vi "BaudDetect-GetDetectArray.vi"(8 "SAM":u8(ring) caption="采样点:" items=["采样一次", "采样三次"], 9 "SJW":u8(ring)=1 caption="同步跳转宽度:" items=["1TQ"=1, "2TQ"=2, "3TQ"=3, "4TQ"=4], 10 "g_data":T2={"b"=-1.0, "e"=-1.0}, 11 "DetectArray in":cluster{"T0":u8, "T1":u8, "br_selfdef":T1}[](array[cluster]) {"br_selfdef"."PHSEG2" items=["CAN_BIT_1TQ"=1, "CAN_BIT_2TQ"=2, "CAN_BIT_3TQ"=3, "CAN_BIT_4TQ"=4, "CAN_BIT_5TQ"=5, "CAN_BIT_6TQ"=6, "CAN_BIT_7TQ"=7, "CAN_BIT_8TQ"=8]; "br_selfdef"."PHSEG1" items=["CAN_BIT_1TQ"=1, "CAN_BIT_2TQ"=2, "CAN_BIT_3TQ"=3, "CAN_BIT_4TQ"=4, "CAN_BIT_5TQ"=5, "CAN_BIT_6TQ"=6, "CAN_BIT_7TQ"=7, "CAN_BIT_8TQ"=8]; "br_selfdef"."PRSEG" items=["CAN_BIT_1TQ"=1, "CAN_BIT_2TQ"=2, "CAN_BIT_3TQ"=3, "CAN_BIT_4TQ"=4, "CAN_BIT_5TQ"=5, "CAN_BIT_6TQ"=6, "CAN_BIT_7TQ"=7, "CAN_BIT_8TQ"=8]; "br_selfdef"."PHS2_SEL" items=["由相位缓冲段1时间指定", "可编程"]; "br_selfdef"."SAM" items=["采样一次", "采样三次"]; "br_selfdef"."BRP" items=["1"=1, "2"=2, "3"=3, "4"=4, "5"=5, "6"=6, "7"=7, "8"=8, "9"=9, "10"=10, "11"=11, "12"=12, "13"=13, "14"=14, "15"=15, "16"=16, "17"=17, "18"=18, "19"=19, "20"=20, "21"=21, "22"=22, "23"=23, "24"=24, "25"=25, "26"=26, "27"=27, "28"=28, "29"=29, "30"=30, "31"=31, "32"=32, "33"=33, "34"=34, "35"=35, "36"=36, "37"=37, "38"=38, "39"=39, "40"=40, "41"=41, "42"=42, "43"=43, "44"=44, "45"=45, "46"=46, "47"=47, "48"=48, "49"=49, "50"=50, "51"=51, "52"=52, "53"=53, "54"=54, "55"=55, "56"=56, "57"=57, "58"=58, "59"=59, "60"=60, "61"=61, "62"=62, "63"=63, "64"=64]; "br_selfdef"."SJW" items=["1TQ"=1, "2TQ"=2, "3TQ"=3, "4TQ"=4]; "br_selfdef"."SYN(nouse)" items=["CAN_BIT_1TQ"=1]}) -> (3 "DetectArray out":cluster{"T0":u8, "T1":u8, "br_selfdef":T1}[](array[cluster]) {"br_selfdef"."PHSEG2" items=["CAN_BIT_1TQ"=1, "CAN_BIT_2TQ"=2, "CAN_BIT_3TQ"=3, "CAN_BIT_4TQ"=4, "CAN_BIT_5TQ"=5, "CAN_BIT_6TQ"=6, "CAN_BIT_7TQ"=7, "CAN_BIT_8TQ"=8]; "br_selfdef"."PHSEG1" items=["CAN_BIT_1TQ"=1, "CAN_BIT_2TQ"=2, "CAN_BIT_3TQ"=3, "CAN_BIT_4TQ"=4, "CAN_BIT_5TQ"=5, "CAN_BIT_6TQ"=6, "CAN_BIT_7TQ"=7, "CAN_BIT_8TQ"=8]; "br_selfdef"."PRSEG" items=["CAN_BIT_1TQ"=1, "CAN_BIT_2TQ"=2, "CAN_BIT_3TQ"=3, "CAN_BIT_4TQ"=4, "CAN_BIT_5TQ"=5, "CAN_BIT_6TQ"=6, "CAN_BIT_7TQ"=7, "CAN_BIT_8TQ"=8]; "br_selfdef"."PHS2_SEL" items=["由相位缓冲段1时间指定", "可编程"]; "br_selfdef"."SAM" items=["采样一次", "采样三次"]; "br_selfdef"."BRP" items=["1"=1, "2"=2, "3"=3, "4"=4, "5"=5, "6"=6, "7"=7, "8"=8, "9"=9, "10"=10, "11"=11, "12"=12, "13"=13, "14"=14, "15"=15, "16"=16, "17"=17, "18"=18, "19"=19, "20"=20, "21"=21, "22"=22, "23"=23, "24"=24, "25"=25, "26"=26, "27"=27, "28"=28, "29"=29, "30"=30, "31"=31, "32"=32, "33"=33, "34"=34, "35"=35, "36"=36, "37"=37, "38"=38, "39"=39, "40"=40, "41"=41, "42"=42, "43"=43, "44"=44, "45"=45, "46"=46, "47"=47, "48"=48, "49"=49, "50"=50, "51"=51, "52"=52, "53"=53, "54"=54, "55"=55, "56"=56, "57"=57, "58"=58, "59"=59, "60"=60, "61"=61, "62"=62, "63"=63, "64"=64]; "br_selfdef"."SJW" items=["1TQ"=1, "2TQ"=2, "3TQ"=3, "4TQ"=4]; "br_selfdef"."SYN(nouse)" items=["CAN_BIT_1TQ"=1]})   [LabVIEW 2011]
uses:
  Baud rate Self Define.ctl
  g_data.ctl
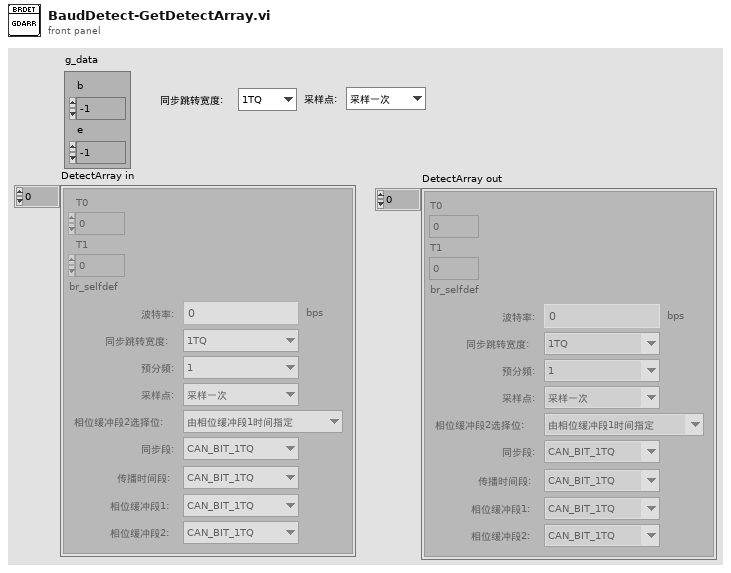
[diagram p1: front panel]
types:
  T1 = typedef "Baud rate Self Define.ctl" = cluster{"BAUD":u32, "SJW":u8, "BRP":u8, "SAM":u8, "PHS2_SEL":u8, "SYN(nouse)":u8, "PRSEG":u8, "PHSEG1":u8, "PHSEG2":u8}
  T2 = typedef "g_data.ctl" = cluster{"b":dbl, "e":dbl}
  T3 = cluster{"BAUD":u32, "簇":cluster{"T0":u8, "T1":u8, "br_selfdef":T1}}
  T4 = cluster{"BAUD":u32, "簇":cluster{"T0":u8, "T1":u8, "br_selfdef":T1}}[]
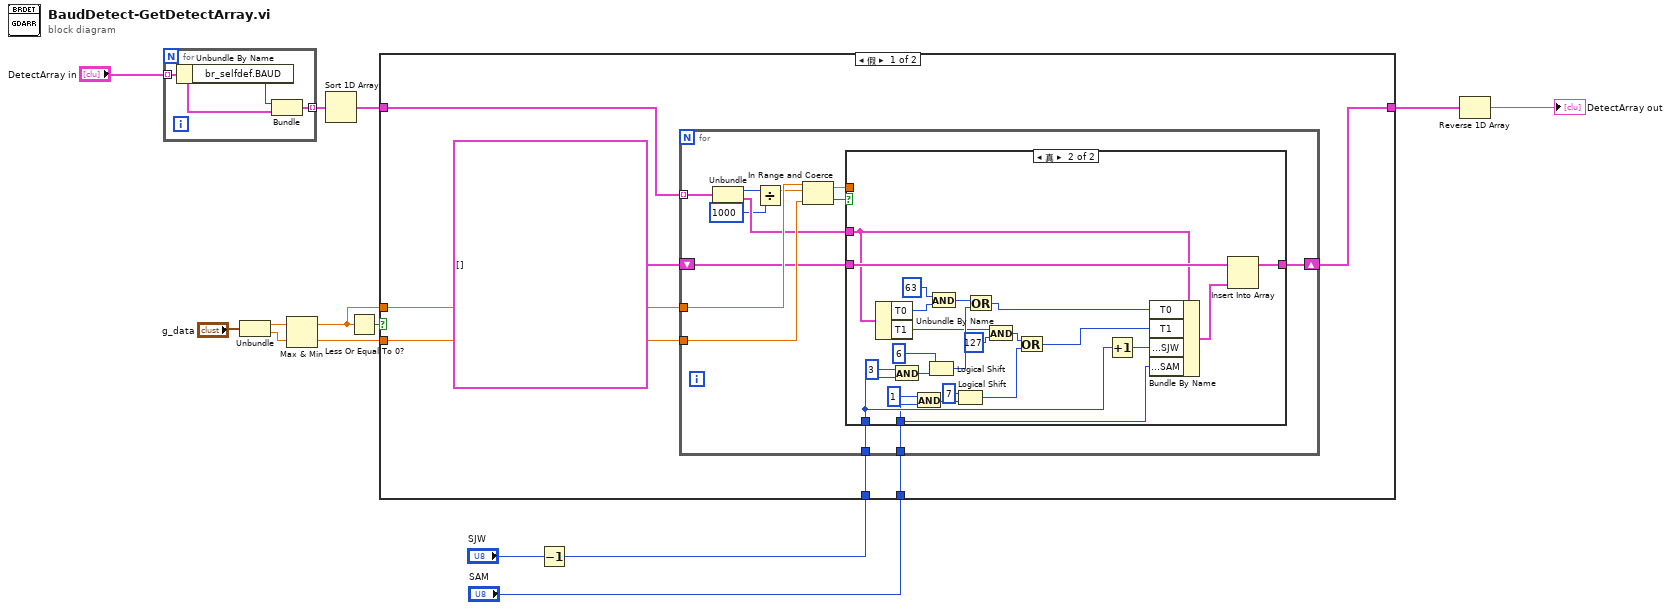
[diagram p0: block diagram]
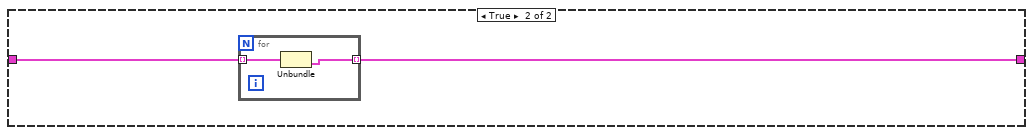
[diagram p3: hidden frame]
diagram:
  n1 = for {
    tunnel: "DetectArray in" -> [w16] mode=indexing
    tunnel: [w15] -> w7 mode=indexing
    n2 = Unbundle By Name(w16) -> ("br_selfdef.BAUD"=w17:u32)
    n3 = Bundle("BAUD"=w17, "簇"=w16) -> (w15:T3)  [unwired: 1 in]
  }
  n4 = Unbundle("g_data") -> ("b"=w13:dbl, "e"=w12:dbl)
  n5 = Max & Min(x=w13, y=w12) -> (max(x,y)=w8:dbl, min(x,y)=w9:dbl)
  n6 = Sort 1D Array(array=w7) -> (sorted array=w5:T4)
  n7 = Less Or Equal To 0?(x=w8) -> (x <= 0?=w11:bool)
  n8 = Decrement(x="SJW") -> (x-1=w3:u8)
  n9 = case shown="假" w11 {
    tunnel: w5 -> [w23 w63]
    tunnel: [w24 w62] -> w10
    tunnel: w9 -> [w20 _]
    tunnel: w8 -> [w21 _]
    tunnel: w3 -> [w19 _]
    tunnel: "SAM" -> [w18 _]
    frame False {
      n10 = for {
        tunnel: w21 -> [w36]
        tunnel: w20 -> [w37]
        shift-right: [w29] -> w24
        shift-left: cluster{"T0":u8, "T1":u8, "br_selfdef":T1}[] [] -> [w30]
        tunnel: w23 -> [w33] mode=indexing
        tunnel: w19 -> [w26]
        tunnel: w18 -> [w25]
        n11 = Unbundle(w33) -> ("BAUD"=w32:u32, "簇"=w31:cluster{"T0":u8, "T1":u8, "br_selfdef":T1})
        n12 = Divide(x=w32, y=u32 1000) -> (x/y=w28:dbl)
        n13 = In Range and Coerce(upper limit=w36, x=w28, lower limit=w37) -> (coerced(x)=w34:dbl, In Range?=w35:bool)
        n14 = case shown="真" w35 {
          tunnel: w34 -> [_ _]
          tunnel: w31 -> [_ w59]
          tunnel: w30 -> [w38 w61]
          tunnel: [w38 w60] -> w29
          tunnel: w26 -> [_ w55]
          tunnel: w25 -> [_ w48]
          frame False {
          }
          frame True {
            n15 = Unbundle By Name(w59) -> ("T0"=w54:u8, "T1"=w44:u8)
            n16 = And(x=u8 3, y=w55) -> (x .and. y?=w49:u8)
            n17 = And(x=u8 1, y=w48) -> (x .and. y?=w46:u8)
            n18 = Logical Shift(y=i8 6, x=w49) -> (x << y=w51:u8)
            n19 = And(x=u8 63, y=w54) -> (x .and. y?=w52:u8)
            n20 = Logical Shift(y=i8 7, x=w46) -> (x << y=w41:u8)
            n21 = Or(x=w52, y=w51) -> (x .or. y?=w50:u8)
            n22 = And(x=w44, y=u8 127 ("x")) -> (x .and. y?=w42:u8)
            n23 = Or(x=w42, y=w41) -> (x .or. y?=w40:u8)
            n24 = Increment(x=w55) -> (x+1=w39:u8)
            n25 = Bundle By Name(cluster=w59, "T0"=w50, "T1"=w40, "br_selfdef.SJW"=w39, "br_selfdef.SAM"=w48) -> (w58:cluster{"T0":u8, "T1":u8, "br_selfdef":T1})
            n26 = Insert Into Array(array=w61, new element=w58) -> (w60:cluster{"T0":u8, "T1":u8, "br_selfdef":T1}[])  [unwired: 1 in]
          }
        }
      }
    }
    frame True {
      n27 = for {
        tunnel: w63 -> [w65] mode=indexing
        tunnel: [w64] -> w62 mode=indexing
        n28 = Unbundle(w65) -> ("簇"=w64:cluster{"T0":u8, "T1":u8, "br_selfdef":T1})  [unwired: 1 out]
      }
    }
  }
  n29 = Reverse 1D Array(array=w10) -> (reversed array=→"DetectArray out":cluster{"T0":u8, "T1":u8, "br_selfdef":T1}[])
